vi "Copy Image Data to Clipboard.vi"(8 "error in (no error)":errorcluster, 11 "image data":T1) -> (0 "error out":errorcluster)   [LabVIEW 2021]
uses:
  <vilib>/picture/picture.llb/imagedata.ctl
  <vilib>/Utility/miscctls.llb/LVBoundsTypeDef.ctl
panel:
  out "2D Picture":picture
  # "This VI needs to open its front panel each time it is called,\nin order for the 2D Picture to be drawn\nFor this reason, the VI runs transparently."
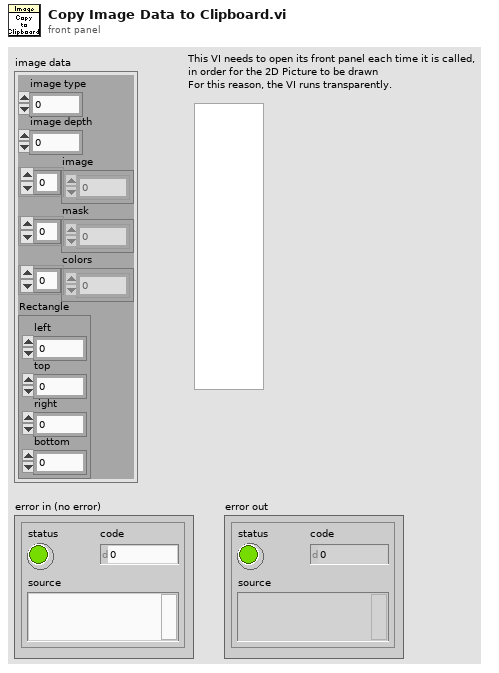
[diagram p1: front panel]
types:
  T1 = typedef "imagedata.ctl" = cluster{"image type":i32, "image depth":i32, "image":u8[], "mask":u8[], "colors":u32[], "Rectangle":cluster{"left":i16, "top":i16, "right":i16, "bottom":i16}}
  T2 = typedef "LVBoundsTypeDef.ctl" = cluster{"Width":u32, "Height":u32}
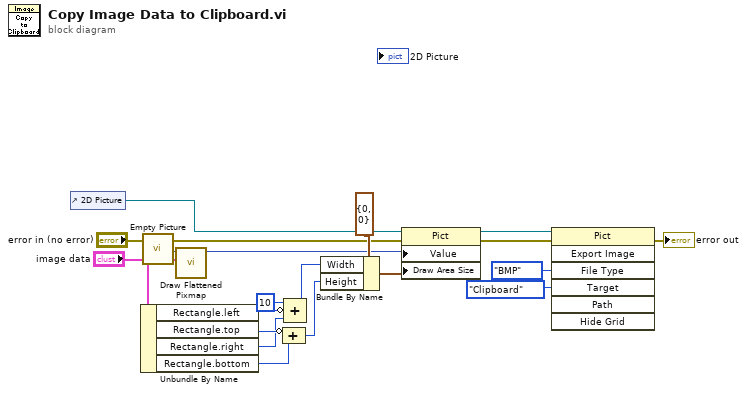
[diagram p0: block diagram]
diagram:
  n1 = control-ref of="2D Picture"() -> (w2:refnum<vi>)
  n2 = Unbundle By Name("image data") -> ("Rectangle.left"=w11:i16, "Rectangle.top"=w16:i16, "Rectangle.right"=w12:i16, "Rectangle.bottom"=w17:i16)
  n3 = call "Empty Picture"() -> ("empty picture"=w6:picture)
  n4 = call <vilib>:"Draw Flattened Pixmap.vi"("image data"="image data", "picture"=w6) -> ("new picture"=w5:picture)  [unwired: 7 in]
  n5 = Compound Arithmetic op=ADD(invert w16, w17) -> (w18:i16)
  n6 = Compound Arithmetic op=ADD(i16 10 ("value"), invert w11, w12) -> (w15:i16)
  n7 = Bundle By Name(cluster=T2 {"Width"=0, "Height"=0} ("Draw Area Size"), "Width"=w15, "Height"=w18) -> (w14:T2)
  n8 = property class="Pict"(reference=w2, error in="error in (no error)", "Value"=w5, "Draw Area Size"=w14) -> (reference out=w9:refnum<vi>, error out=w7:errorcluster)
  n9 = invoke class="Pict" method="Export Image"(reference=w9, error in=w7, "File Type"=enum32{"BMP", "EPS", "EMF", "PICT"}."BMP", "Target"=enum32{"File", "Clipboard"}."Clipboard") -> (error out=→"error out":errorcluster)  [unwired: 3 in, 6 out]
